vi "overlay3channels.vi"(8 "RGB Overlay":T2, 11 "Array":T1(array[cluster])) -> ()   [LabVIEW 2012]
uses:
  <vilib>/vision/Image Controls.llb/IMAQ Image.ctl
  Custom Controls/Ch selector.ctl
  <vilib>/vision/NI_Vision_Development_Module.lvlib
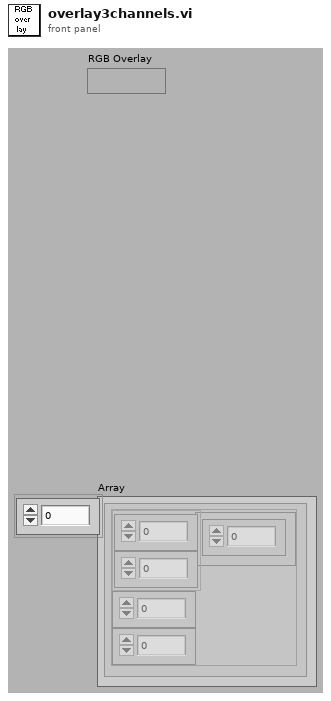
[diagram p1: front panel]
types:
  T1 = cluster{"Array":i16[][], "Numeric Control":i32, "Numeric Control":i32}[]
  T2 = typedef "IMAQ Image.ctl" = refnum<image>
  T3 = typedef "Ch selector.ctl" = enum16{"none", "Ch 1", "Ch 2", "Ch 3", "Ch 4", "Ch 5"}
  T4 = cluster{"Array":i16[][], "Numeric Control":i32, "Numeric Control":i32}
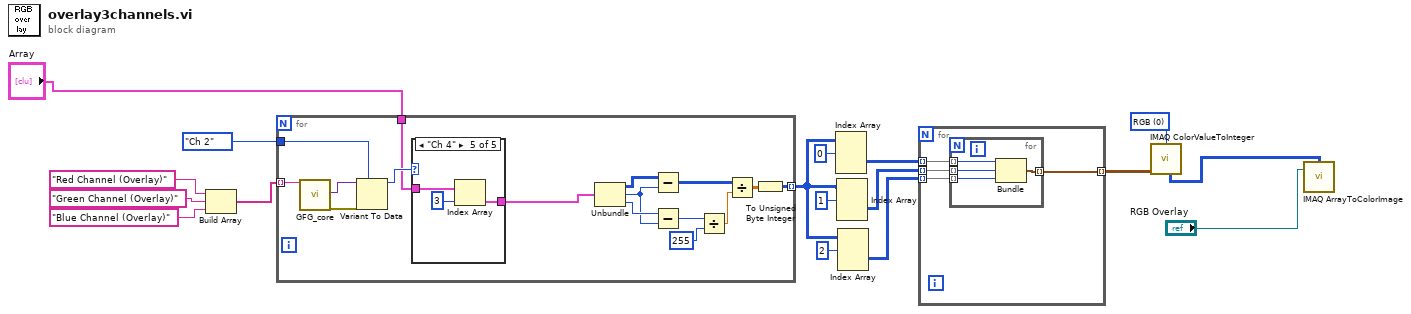
[diagram p0: block diagram]
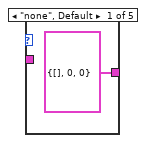
[diagram p2: hidden frame]
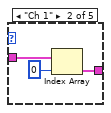
[diagram p3: hidden frame]
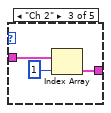
[diagram p4: hidden frame]
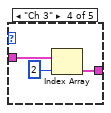
[diagram p5: hidden frame]
diagram:
  w16 = u16 0 items=["RGB", "HSL", "HSV", "HSI"] ("Color Mode")
  n1 = Build Array("Red Channel (Overlay)" ("Variable Name in"), "Green Channel (Overlay)" ("Variable Name in"), "Blue Channel (Overlay)" ("Variable Name in")) -> (w10:string[])
  n2 = for {
    tunnel: w10 -> [w33] mode=indexing
    tunnel: Ch_selector."Ch 2" ("Red Channel (Overlay)") -> [w31]
    tunnel: "Array" -> [w28]
    tunnel: [w19] -> w5 mode=indexing
    n3 = call "GFG_core.vi"("Variable Name in"=w33) -> ("Variant Out"=w30:variant, "error out"=w32:errorcluster)  [unwired: 12 in, 5 out]
    n4 = Variant To Data(error in=w32, type=w31, Variant=w30) -> (data=w29:T3)  [unwired: 1 out]
    n5 = case shown="\"Ch 4\"" w29 {
      tunnel: w28 -> [_ w37 w40 w43 w46]
      tunnel: [cluster{i16[][], i32, i32} {[], 0, 0} w35 w38 w41 w44] -> w27
      frame "none", Default {
      }
      frame "Ch 1" {
        n6 = Index Array(array=w37, index=0) -> (element=w35:T4)
      }
      frame "Ch 2" {
        n7 = Index Array(array=w40, index=1) -> (element=w38:T4)
      }
      frame "Ch 3" {
        n8 = Index Array(array=w43, index=2) -> (element=w41:T4)
      }
      frame "Ch 4" {
        n9 = Index Array(array=w46, index=3) -> (element=w44:T4)
      }
    }
    n10 = Unbundle(w27) -> ("Array"=w22:i16[][], "Numeric Control"=w18:i32, "Numeric Control"=w21:i32)
    n11 = Subtract(x=w22, y=w18) -> (x-y=w25:i32[][])
    n12 = Subtract(x=w21, y=w18) -> (x-y=w26:i32)
    n13 = Divide(x=w26, y=i16 255) -> (x/y=w24:dbl)
    n14 = Divide(x=w25, y=w24) -> (x/y=w20:dbl[][])
    n15 = To Unsigned Byte Integer(number=w20) -> (unsigned 8bit integer=w19:u8[][])
  }
  n16 = Index Array(array=w5, index (dim 0)=0 ("index (page)")) -> (element=w3:u8[][])  [unwired: 2 in]
  n17 = Index Array(array=w5, index (dim 0)=1 ("index (page)")) -> (element=w2:u8[][])  [unwired: 2 in]
  n18 = Index Array(array=w5, index (dim 0)=2 ("index (page)")) -> (element=w1:u8[][])  [unwired: 2 in]
  n19 = for {
    tunnel: w3 -> [w48] mode=indexing
    tunnel: [w50] -> w17 mode=indexing
    tunnel: w1 -> [w49] mode=indexing
    tunnel: w2 -> [w47] mode=indexing
    n20 = for {
      tunnel: w48 -> [w54] mode=indexing
      tunnel: [w53] -> w50 mode=indexing
      tunnel: w49 -> [w52] mode=indexing
      tunnel: w47 -> [w51] mode=indexing
      n21 = Bundle(w54, w51, w52) -> (w53:cluster{u8, u8, u8})  [unwired: 1 in]
    }
  }
  n22 = call "IMAQ ColorValueToInteger"("2D Color value array"=w17, "Color Mode"=w16) -> ("2D U32 array"=w15:u32[][])  [unwired: 3 in, 3 out]
  n23 = call "IMAQ ArrayToColorImage"("Image Pixels (U32)"=w15, "Image"="RGB Overlay") -> ()  [unwired: 3 in, 2 out]
